vi "禹山电导率校准.vi"() -> ()   [LabVIEW 2016, in "斯坦道多参数.lvlib"]
uses:
  <vilib>/Utility/miscctls.llb/LVPointTypeDef.ctl
  <vilib>/Analysis/NI_AALBase.lvlib
  <vilib>/Analysis/NI_AALPro.lvlib
  <vilib>/Utility/config.llb/NI_LVConfig.lvlib
panel:
  out "盐度":dbl caption="盐度测量值" format="%#.2f"
  out "通讯状态":string
  out "第二点校准值":dbl
  out "第一点校准值":dbl
  out "最小值":sgl format="%.2g"
  out "最大值":sgl format="%.2g"
  in  "校准停止":bool
  in  "校准模式":u16(ring) items=["两点校准", "单点校准"]
  in  "标液2":dbl
  in  "标液1":dbl
  out "波形图表":sgl(graph) caption="历史曲线"
  out "温度测量值":dbl caption="温度" format="%#.2f"
  out "变异系数":dbl format="%.6g"
  out "standard deviation":dbl caption="标准差" format="%0.2f"
  out "mean":dbl caption="均值" format="%0.2f"
  out "提示":string
  in  "校准启动":bool
  out "测试值":dbl format="%#.2f"
  out "电极斜率":dbl format="%#.6f"
  out "电极零点":dbl format="%#.6f"
  # "电导率电极设定"
  # "℃"
  # "μS/cm"
  # "ppt"
  # "请选择校准模式:"
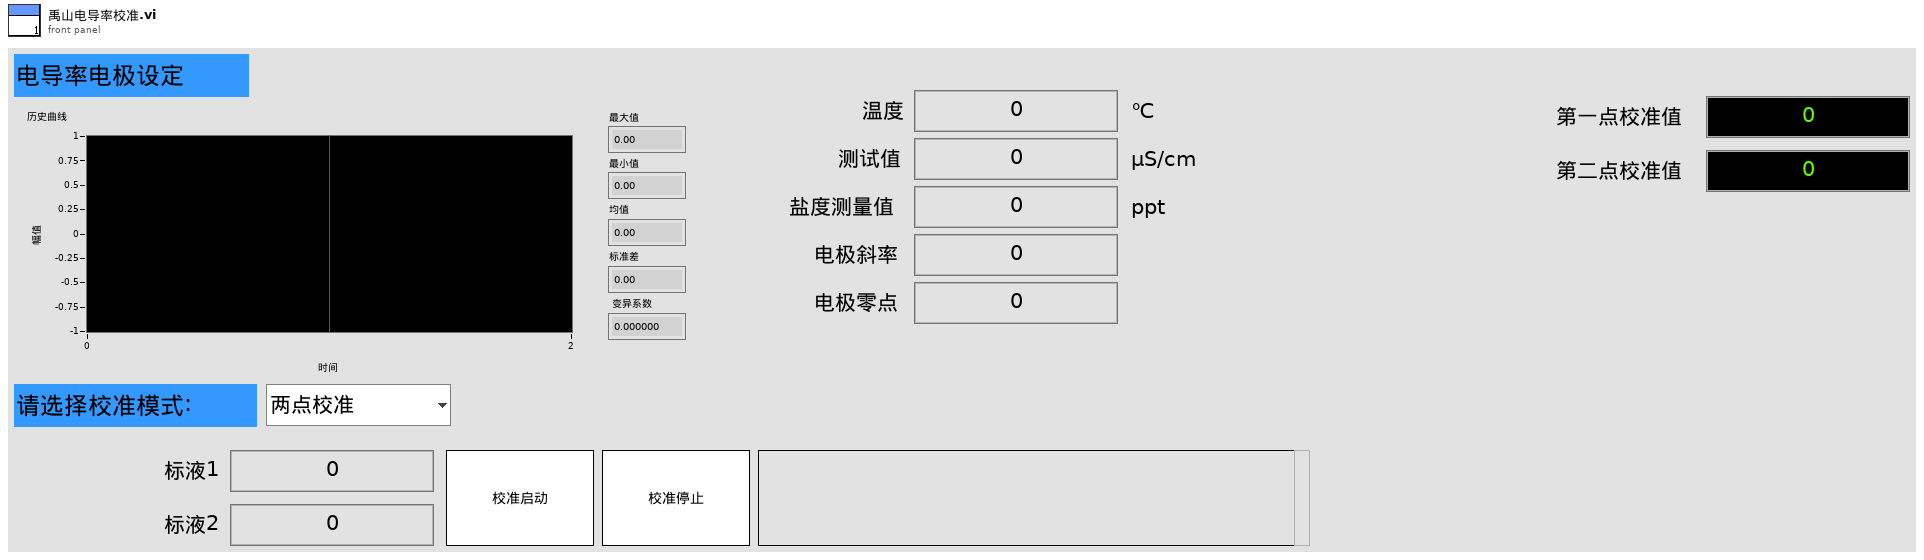
[diagram p1: front panel]
types:
  T1 = typedef "LVPointTypeDef.ctl" = cluster{"Horizontal":i16, "Vertical":i16}
  T2 = typedef "NI_LVConfig.lvlib/Config Data RefNum.ctl" = refnum<k1>
  T3 = cluster{"温度测量值":sgl, "测量值":sgl, "温度偏移修正值":sgl, "信号值":sgl}
  T4 = enum8{"Enabled", "Disabled", "Disabled and Grayed Out"}
  T5 = cluster{"ph":bool, "DO":bool, "Cond":bool, "Turb":bool, "叶绿素a":bool, "藻密度":bool, "ORP":bool}
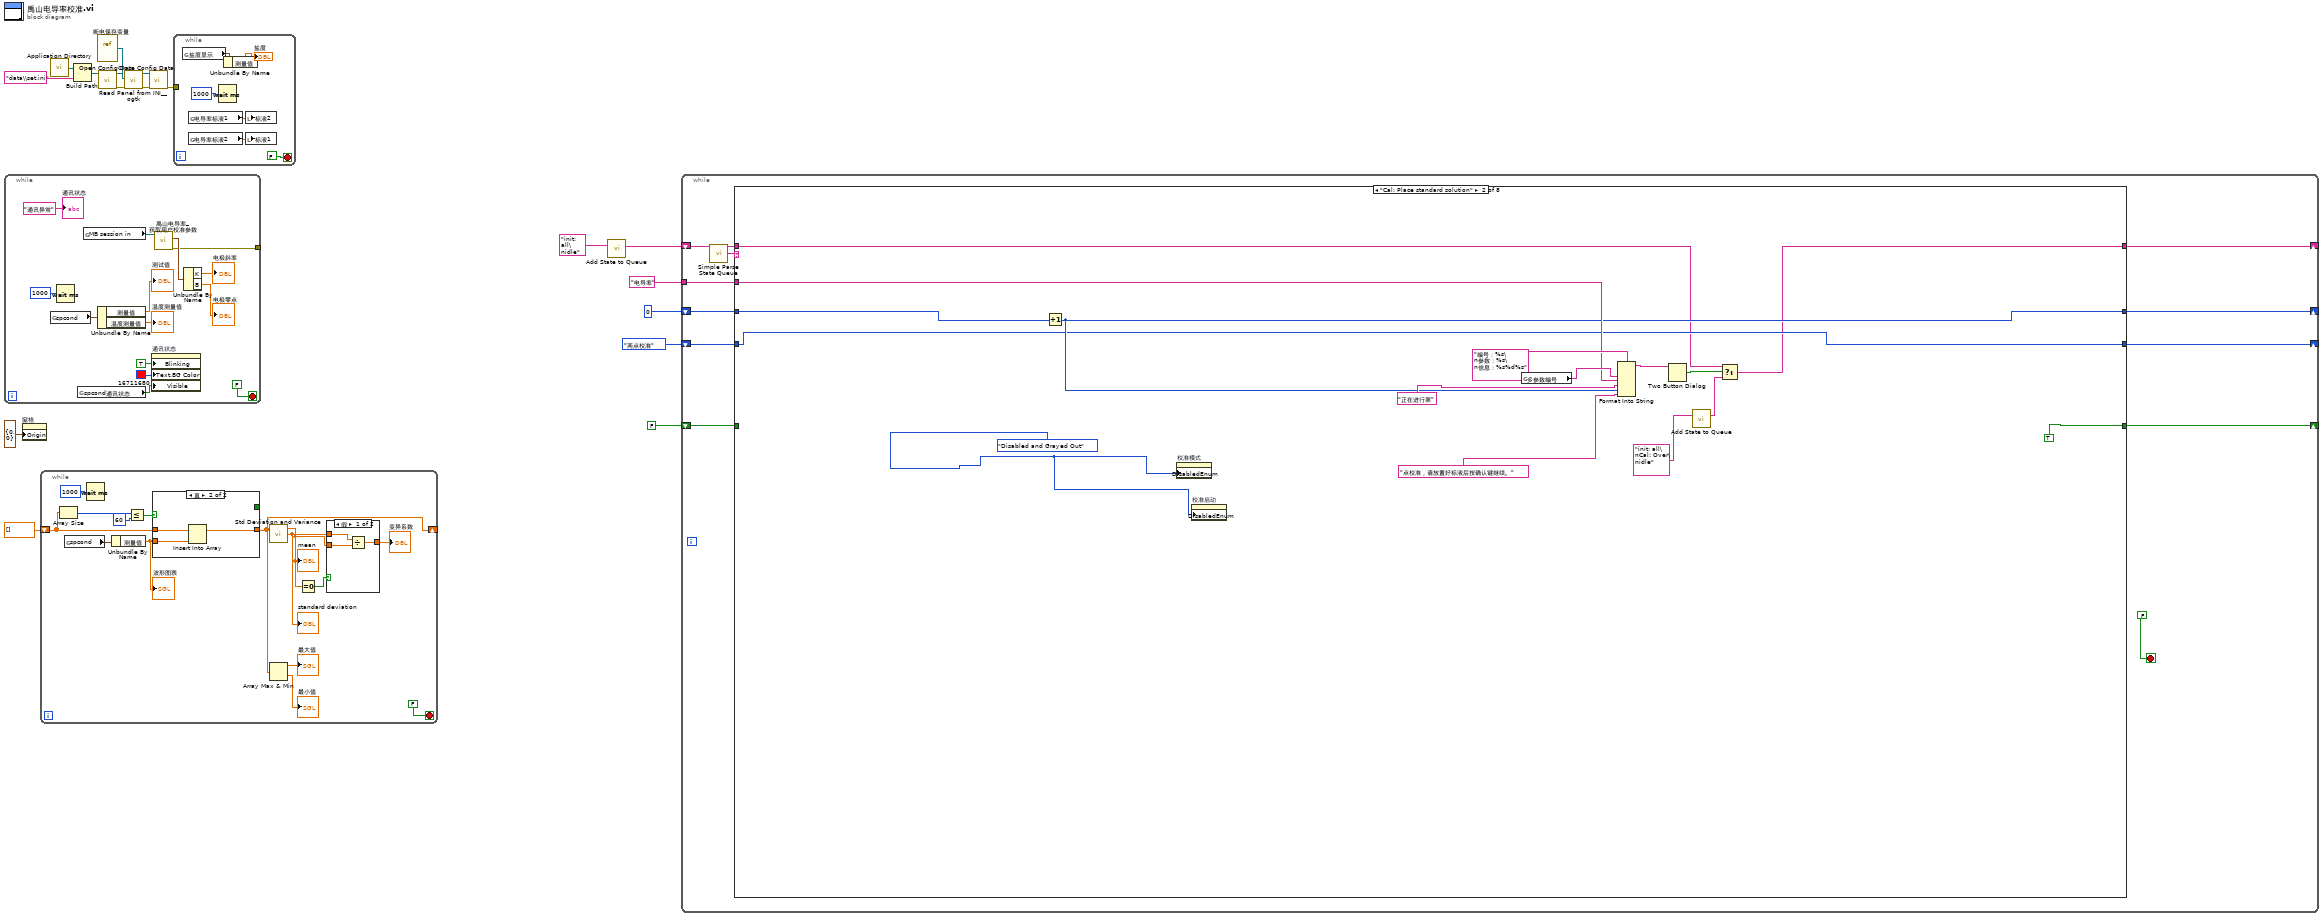
[diagram p0: block diagram]
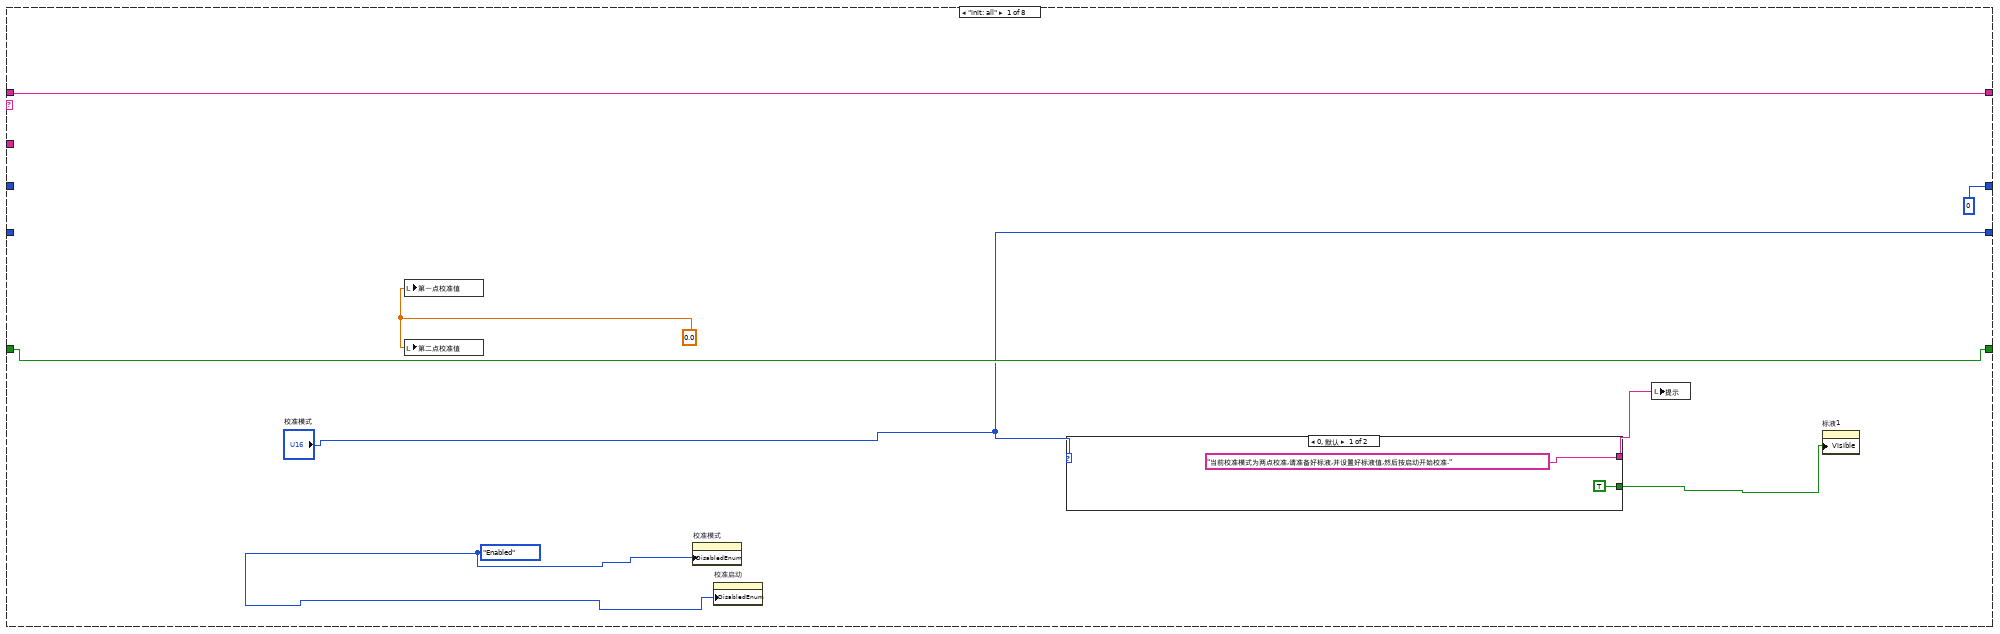
[diagram p2: hidden frame]
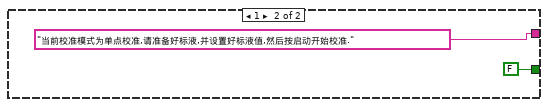
[diagram p3: hidden frame]
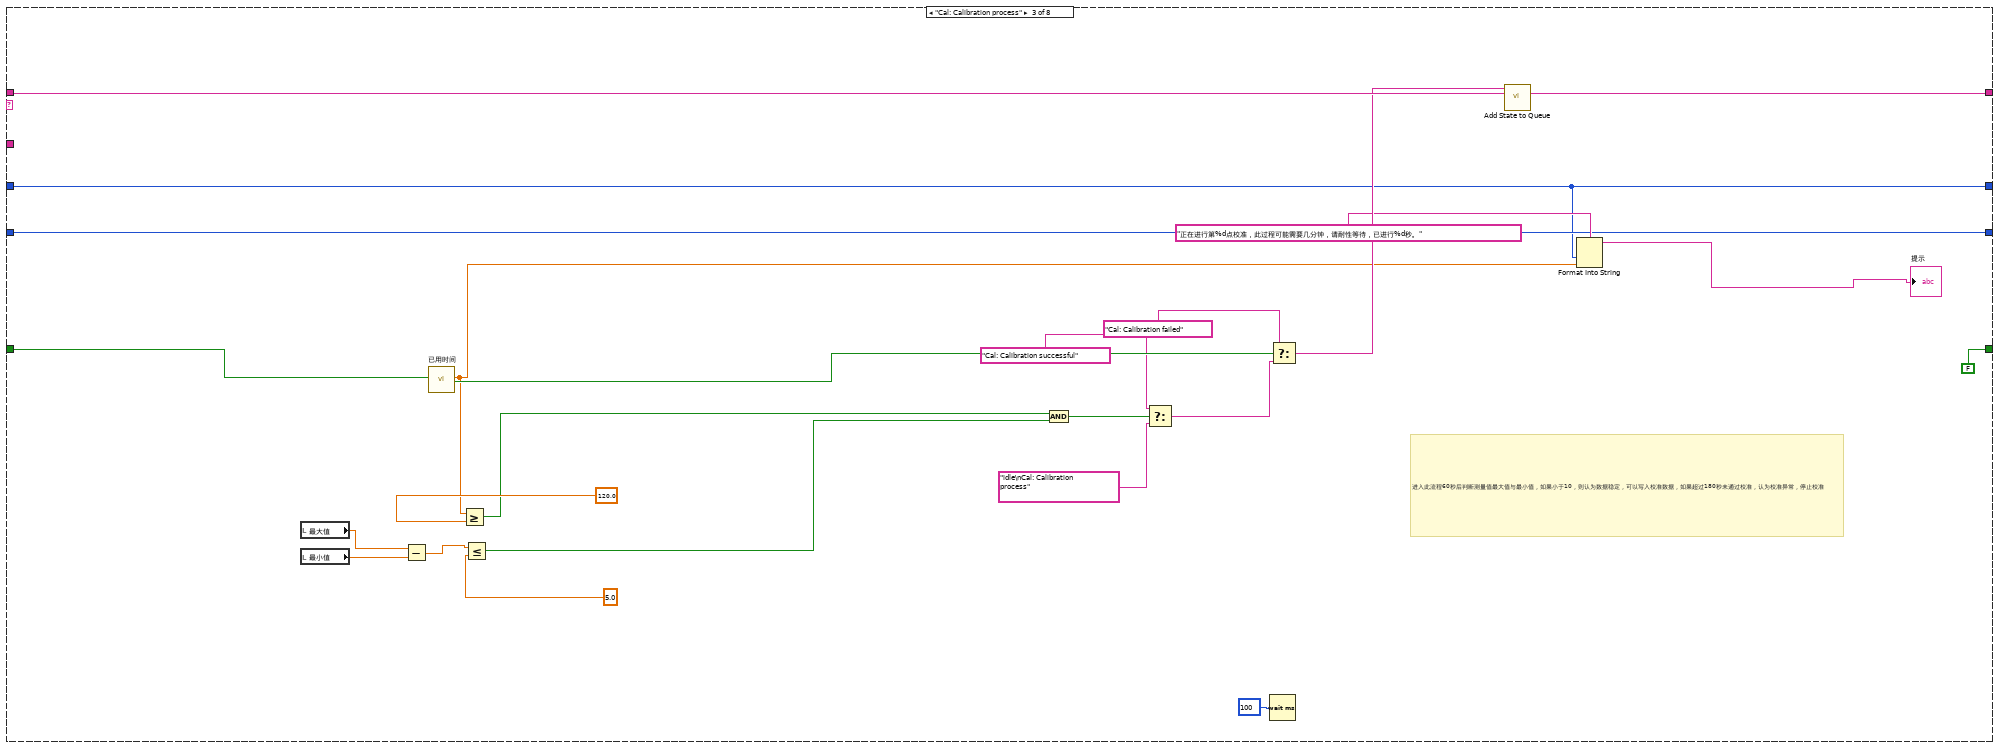
[diagram p4: hidden frame]
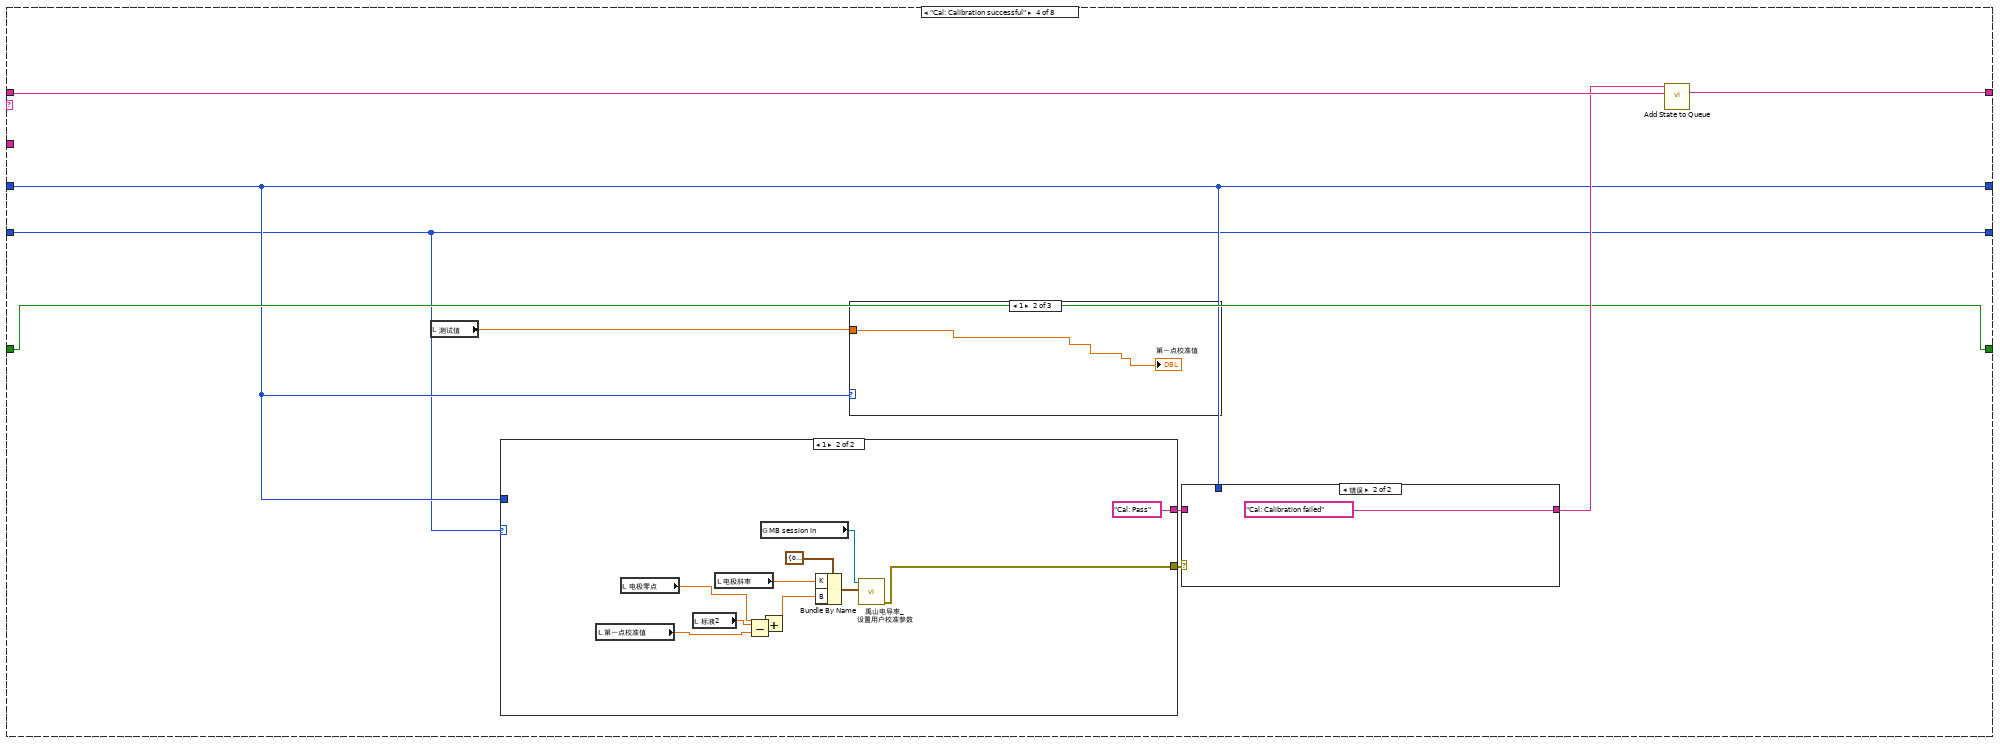
[diagram p5: hidden frame]
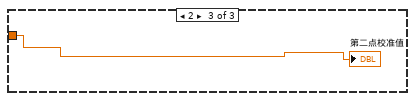
[diagram p7: hidden frame]
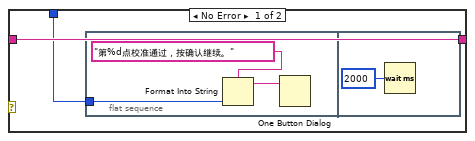
[diagram p8: hidden frame]
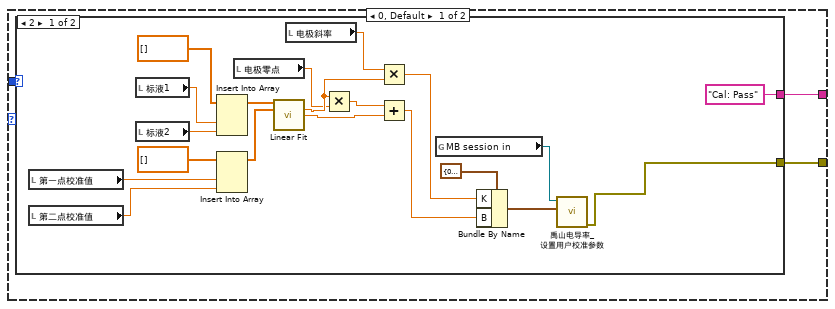
[diagram p9: hidden frame]
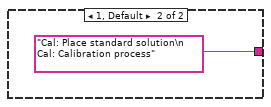
[diagram p10: hidden frame]
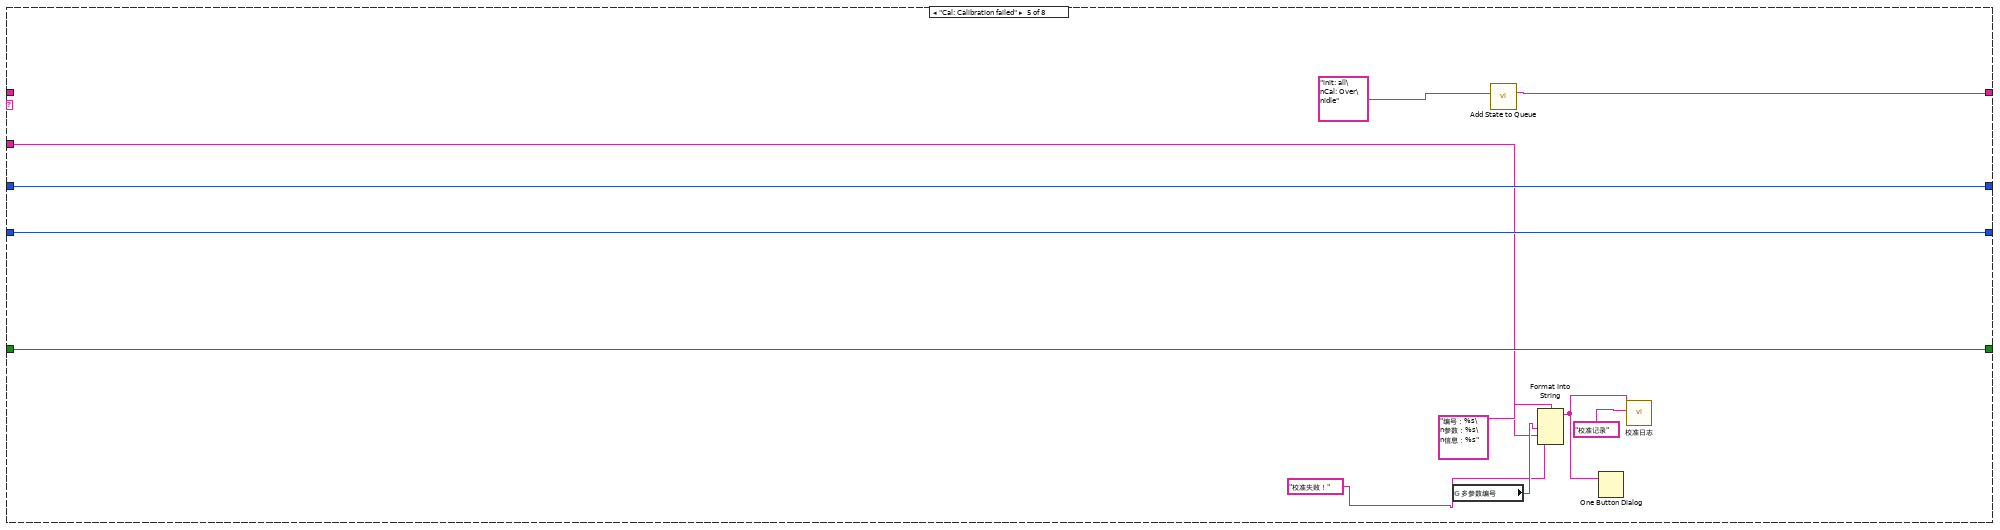
[diagram p11: hidden frame]
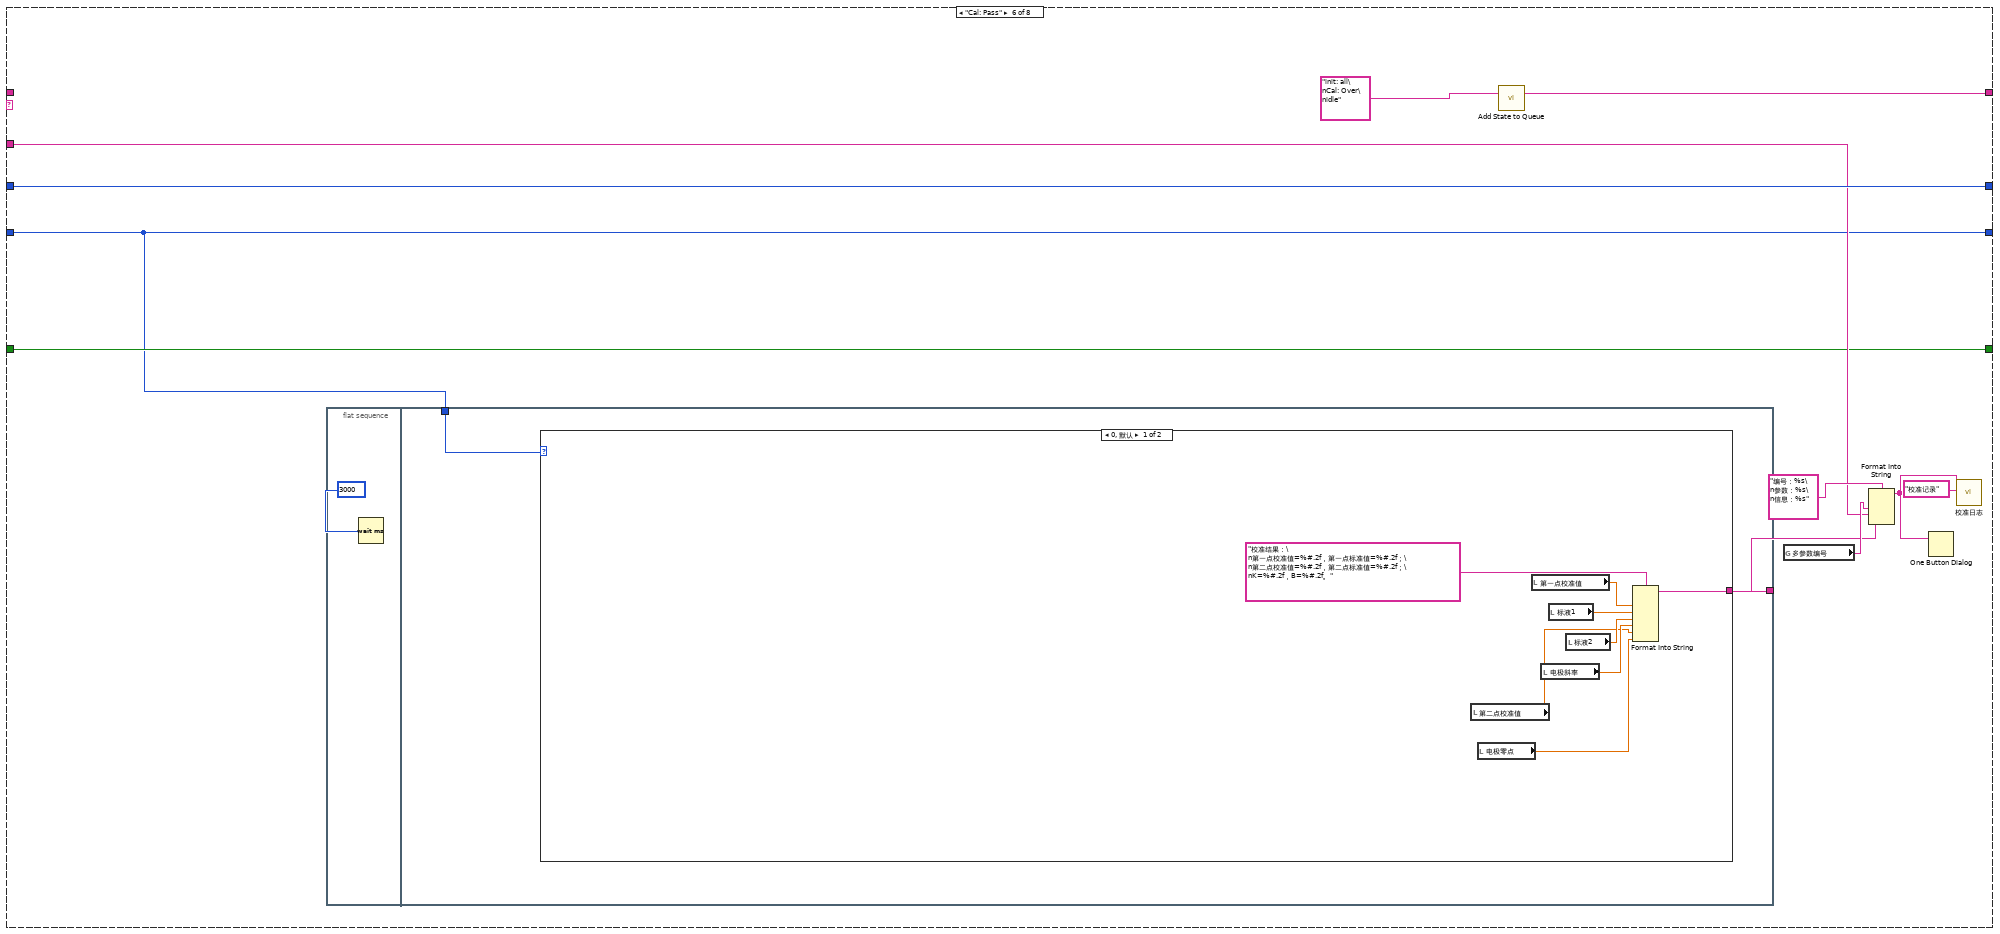
[diagram p12: hidden frame]
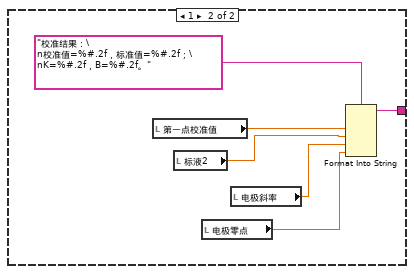
[diagram p13: hidden frame]
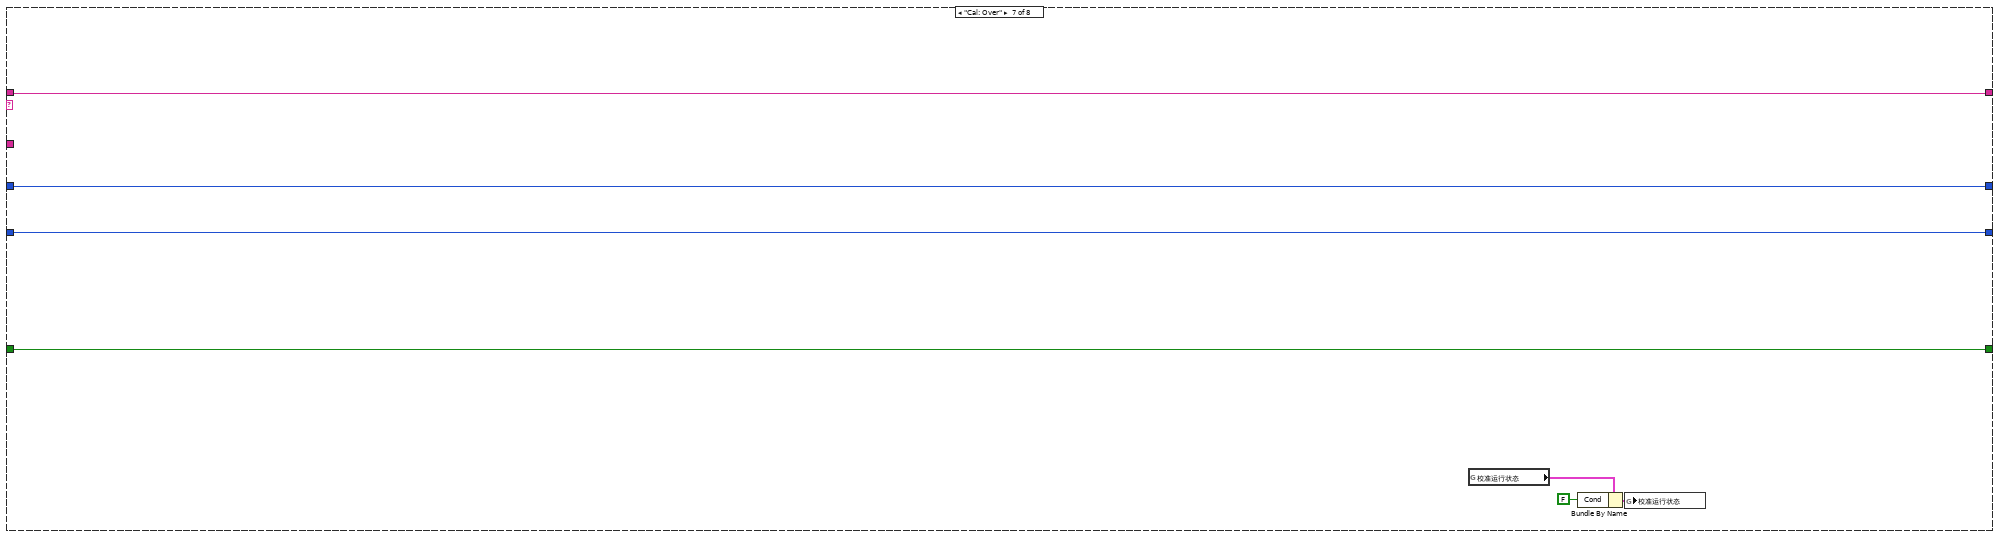
[diagram p14: hidden frame]
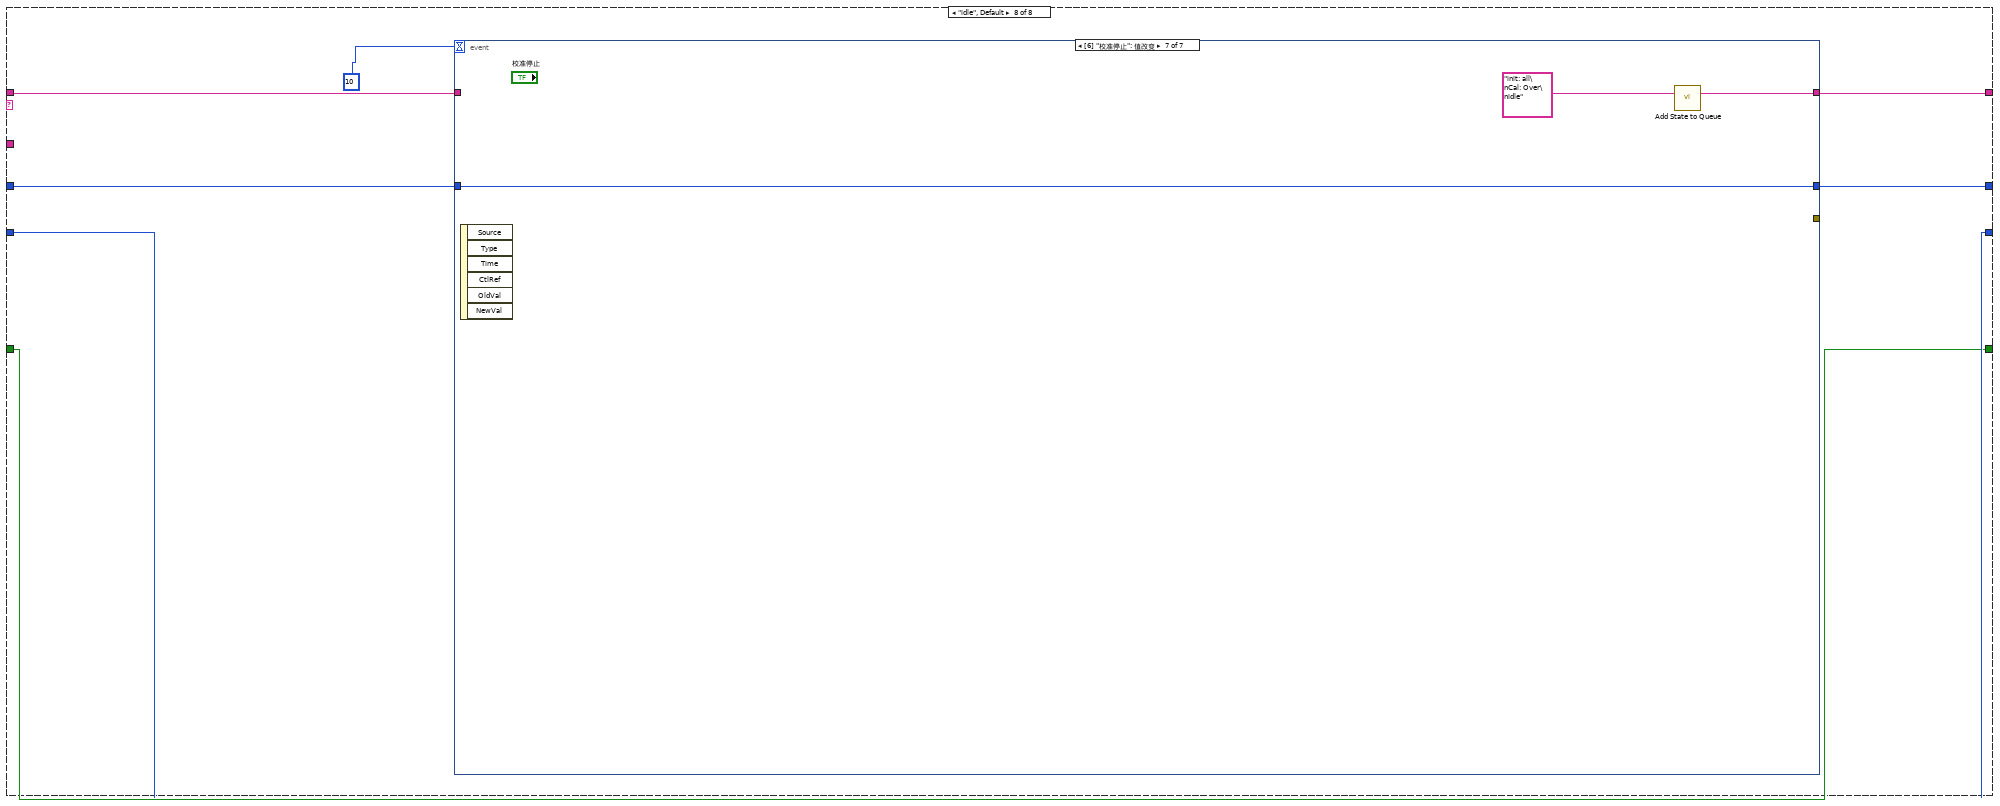
[diagram p15: hidden frame]
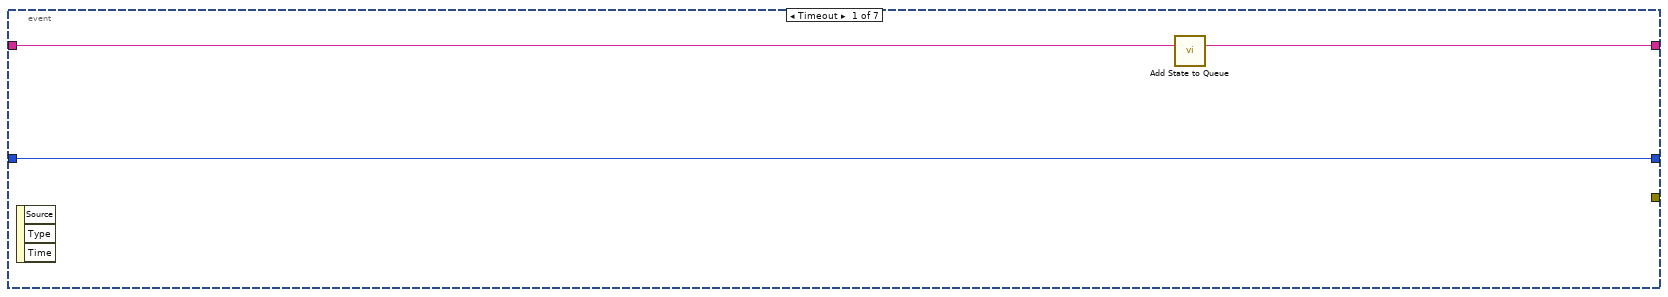
[diagram p16: hidden frame]
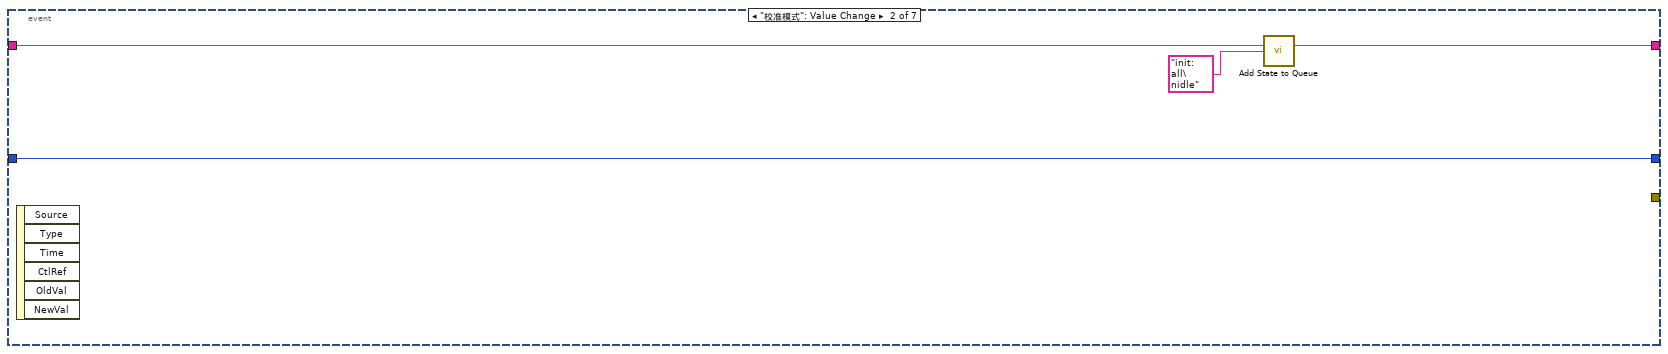
[diagram p17: hidden frame]
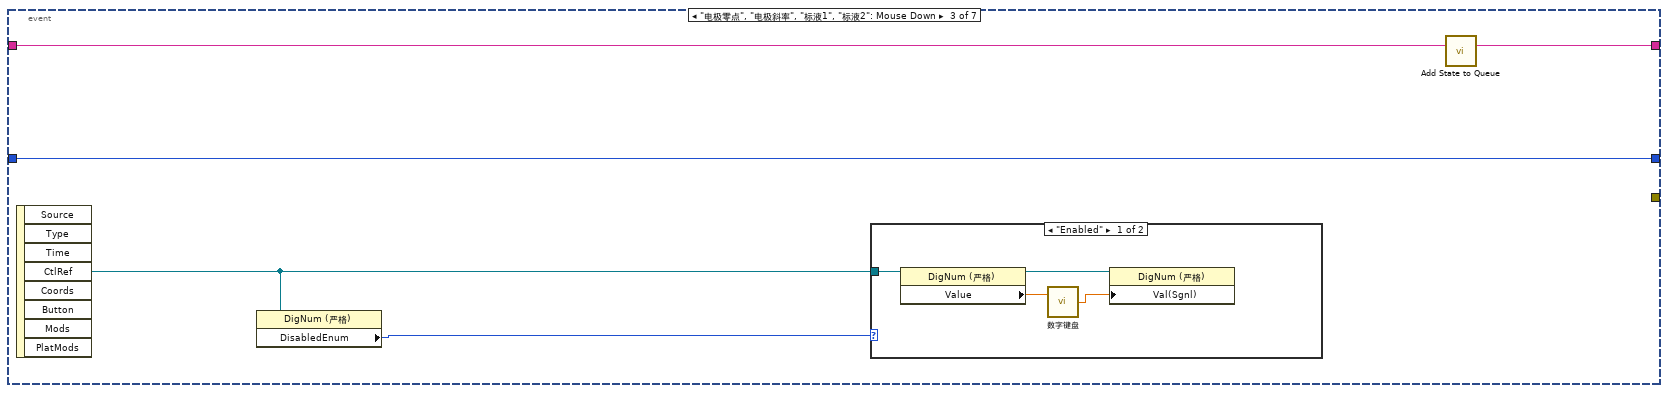
[diagram p18: hidden frame]
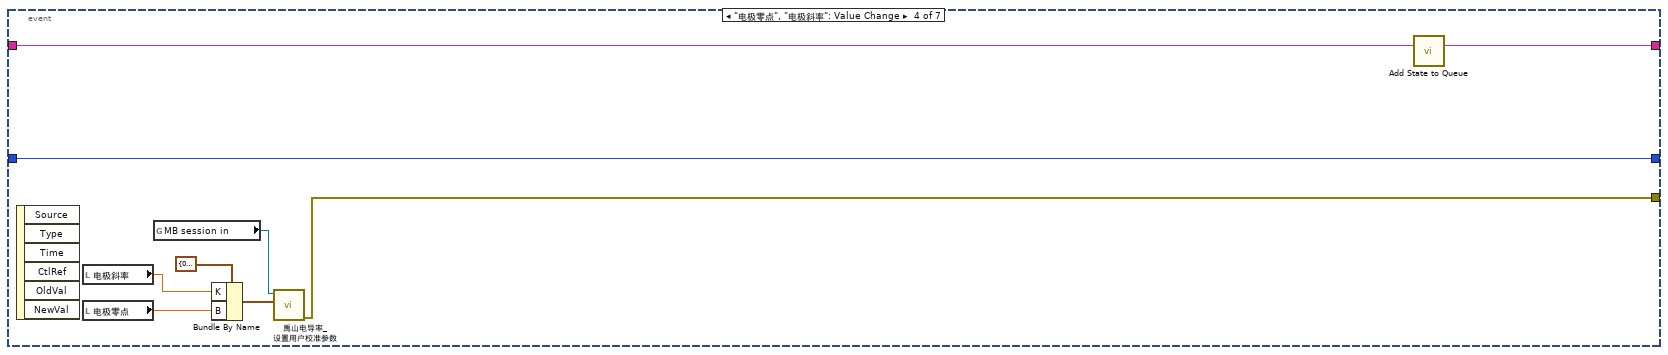
[diagram p20: hidden frame]
diagram:
  n1 = while {
    tunnel: [w26] -> _
    stop <- FALSE stop-if-true
    n2 = global read "禹山过程全局变量.vi" "spcond"() -> (w23:cluster{"温度测量值":sgl, "测量值":sgl, "错误标志":u16})
    n3 = Wait (ms)(milliseconds to wait=u32 1000 ("等待时间（毫秒）")) -> ()  [unwired: 1 out]
    n4 = global read "多参数全局变量.vi" "spcond通讯状态"() -> (w18:bool)
    n5 = global read "多参数全局变量.vi" "MB session in"() -> (w22:refnum<class "MB_Master.lvclass">)
    n6 = Unbundle By Name(w23) -> ("测量值"=→"测试值":sgl, "温度测量值"=→"温度测量值":sgl)
    n7 = property on="通讯状态" class="Str"("Blinking"=TRUE ("闪烁"), "Text.BG Color"=u32 16711680, "Visible"=w18) -> ()  [unwired: 2 in, 2 out]
    n8 = call "禹山电导率_获取用户校准参数.vi"("MB session in"=w22) -> ("error out"=w26:errorcluster, "输出值"=w29:cluster{"K":sgl, "B":sgl})  [unwired: 8 in, 1 out]
    n9 = Unbundle By Name(w29) -> ("K"=→"电极斜率":sgl, "B"=→"电极零点":sgl)
    "通讯状态" <- "通讯异常" ("当前串口")
  }
  n10 = property on="窗格" class="Pane"("Origin"=T1 {"Horizontal"=0, "Vertical"=0} ("原点")) -> ()  [unwired: 2 in, 2 out]
  n11 = while {
    shift-right: [w34] -> _
    shift-left: sgl[] [] -> [w42]
    stop <- FALSE stop-if-true
    n12 = Array Size(array=w42) -> (size(s)=w44:i32)
    n13 = global read "禹山过程全局变量.vi" "spcond"() -> (w36:cluster{"温度测量值":sgl, "测量值":sgl, "错误标志":u16})
    n14 = Wait (ms)(milliseconds to wait=u32 1000 ("等待时间（毫秒）")) -> ()  [unwired: 1 out]
    n15 = Unbundle By Name(w36) -> ("测量值"=w35:sgl)
    "波形图表" <- w35
    n16 = Less Or Equal?(x=w44, y=60) -> (x <= y?=w43:bool)
    n17 = case shown="真" w43 {
      tunnel: w42 -> [w55 w58]
      tunnel: w35 -> [w53 w57]
      tunnel: [w51 w56] -> w34
      tunnel: [TRUE _] -> _
      frame False {
        n18 = Replace Array Subset(array=w55, new element=w53) -> (w54:sgl[])  [unwired: 1 in]
        n19 = Rotate 1D Array(1:w54, 2:-1 ("n")) -> (0:w51:sgl[])
      }
      frame True {
        n20 = Insert Into Array(array=w58, new element=w57) -> (w56:sgl[])  [unwired: 1 in]
      }
    }
    n21 = call <vilib>:"Std Deviation and Variance.vi"("X"=w34) -> ("mean"=w37:dbl, "standard deviation"=w38:dbl)  [unwired: 1 in, 1 out]
    "standard deviation" <- w38
    "mean" <- w37
    n22 = Array Max & Min(array=w34) -> (max value=→"最大值":sgl, min value=→"最小值":sgl)  [unwired: 2 out]
    n23 = Equal To 0?(x=w37) -> (x = 0?=w41:bool)
    n24 = case shown="假" w41 {
      tunnel: w38 -> [w49 _]
      tunnel: [w48 _] -> w40
      tunnel: w37 -> [w47 _]
      frame False {
        n25 = Divide(x=w49, y=w47) -> (x/y=w48:dbl)
      }
      frame True {
      }
    }
    "变异系数" <- w40
  }
  n26 = call <vilib>:"Application Directory.vi"() -> ("Application Directory"=w12:path)
  n27 = Build Path(base path=w12, name or relative path="data\\set.ini" ("名称或相对路径")) -> (appended path=w13:path)
  n28 = vi-ref "断电保存变量.vi"() -> (w15:refnum<vi>)
  n29 = call <vilib>:"Open Config Data.vi"("configuration file path"=w13) -> ("error out"=w9:errorcluster, "refnum"=w8:T2)  [unwired: 8 in, 1 out]
  n30 = call <userlib>:"Read Panel from INI__ogtk.vi"("error in (no error)"=w9, "VI ref"=w15, "refnum"=w8) -> ("error out"=w11:errorcluster, "refnum out"=w10:T2)  [unwired: 7 in]
  n31 = call <vilib>:"Close Config Data.vi"("error in (no error)"=w11, "refnum"=w10) -> ("error out"=w7:errorcluster)  [unwired: 8 in, 1 out]
  n32 = while {
    tunnel: w7 -> [_]
    stop <- FALSE stop-if-true
    n33 = global read "多参数全局变量.vi" "盐度显示"() -> (w60:T3)
    n34 = global read "断电保存变量.vi" "电导率标液1"() -> (w61:dbl)
    n35 = global read "断电保存变量.vi" "电导率标液2"() -> (w62:dbl)
    n36 = Wait (ms)(milliseconds to wait=u32 1000 ("等待时间（毫秒）")) -> ()  [unwired: 1 out]
    n37 = Unbundle By Name(w60) -> ("测量值"=→"盐度":sgl)
    n38 = local write "标液2"(w61) -> ()
    n39 = local write "标液1"(w62) -> ()
  }
  n40 = call "Add State to Queue.vi"("State(s) In (\"\")"="init: all\nidle" ("State(s) In (\"\")")) -> ("States Out"=w5:string)  [unwired: 14 in]
  n41 = while {
    shift-right: [w72] -> _
    shift-left: w5 -> [w76]
    shift-right: [w69] -> _
    shift-left: 0 -> [w71]
    tunnel: "电导率" ("State(s) In (\"\")") -> [w70]
    shift-right: [w67] -> _
    shift-left: enum16{"两点校准", "单点校准"}."两点校准" ("校准模式") -> [w68]
    shift-right: [w65] -> _
    shift-left: FALSE -> [w66]
    stop <- FALSE stop-if-true
    n42 = call "Simple Parse State Queue.vi"("State Queue"=w76) -> ("Remain States"=w73:string, "Next State"=w74:string)  [unwired: 13 in]
    n43 = case shown="\"Cal: Place standard solution\"" w74 {
      tunnel: w73 -> [w84 w92 w123 w135 _ _ w224 w234]
      tunnel: [w84 w91 w122 w134 w189 w194 w224 w233] -> w72
      tunnel: w71 -> [_ w100 w107 w130 w192 w203 w223 w231]
      tunnel: w70 -> [_ w101 _ _ w183 w199 _ _]
      tunnel: [0 w98 w107 w130 w192 w203 w223 w232] -> w69
      tunnel: w68 -> [_ w97 w108 w129 w191 w195 w222 w230]
      tunnel: ["校准模式" w97 w108 w129 w191 w195 w222 w230] -> w67
      tunnel: w66 -> [w81 _ w110 w131 w190 w198 w221 w228]
      tunnel: [w81 TRUE FALSE w131 w190 w198 w221 w228] -> w65
      frame "init: all" {
        w78 = T4."Enabled" ("禁用")
        w80 = 0.0 ("第一点校准值")
        n44 = local write "第一点校准值"(w80) -> ()
        n45 = local write "第二点校准值"(w80) -> ()
        n46 = property on="校准模式" class="Ring (严格)"("DisabledEnum"=w78) -> ()  [unwired: 2 in, 2 out]
        n47 = property on="校准启动" class="Bool"("DisabledEnum"=w78) -> ()  [unwired: 2 in, 2 out]
        n48 = case shown="0, 默认" "校准模式" {
          tunnel: ["当前校准模式为两点校准,请准备好标液,并设置好标液值,然后按启动开始校准." ("提示") "当前校准模式为单点校准,请准备好标液,并设置好标液值,然后按启动开始校准." ("提示")] -> w83
          tunnel: [TRUE ("可见") FALSE ("可见")] -> w77
          frame 0, Default {
          }
          frame 1 {
          }
        }
        n49 = local write "提示"(w83) -> ()
        n50 = property on="标液1" class="DigNum (严格)"("Visible"=w77) -> ()  [unwired: 2 in, 2 out]
      }
      frame "Cal: Place standard solution" {
        w90 = T4."Disabled and Grayed Out" ("禁用")
        n51 = Increment(x=w100) -> (x+1=w98:i32)
        n52 = property on="校准模式" class="Ring (严格)"("DisabledEnum"=w90) -> ()  [unwired: 2 in, 2 out]
        n53 = property on="校准启动" class="Bool"("DisabledEnum"=w90) -> ()  [unwired: 2 in, 2 out]
        n54 = global read "多参数全局变量.vi" "多参数编号"() -> (w103:string)
        n55 = Format Into String(format string="编号：%s\n参数：%s\n信息：%s%d%s" ("格式字符串"), w103, w101, "正在进行第" ("消息"), w98, "点校准，请放置好标液后按确认键继续。" ("消息")) -> (resulting string=w95:string)  [unwired: 2 in, 1 out]
        n56 = Two Button Dialog(message=w95) -> (T button?=w94:bool)  [unwired: 2 in]
        n57 = call "Add State to Queue.vi"("State(s) In (\"\")"="init: all\nCal: Over\nidle" ("State(s) In (\"\")")) -> ("States Out"=w93:string)  [unwired: 14 in]
        n58 = Select(t=w92, s=w94, f=w93) -> (s? t:f=w91:string)
      }
      frame "Cal: Calibration process" {
        # "进入此流程60秒后判断测量值最大值与最小值，如果小于10，则认为数据稳定，可以写入校准数据，如果超过180秒未通过校准，认为校准异常，停止校准"
        n59 = local read "最大值"() -> (w127:sgl)
        n60 = local read "最小值"() -> (w126:sgl)
        n61 = Subtract(x=w127, y=w126) -> (x-y=w128:sgl)
        n62 = call "已用时间"("Reset"=w110) -> ("Elapsed Time (s)"=w106:dbl, "Time has Elapsed"=w124:bool)  [unwired: 11 in, 6 out]
        n63 = Greater Or Equal?(x=w106, y=120.0) -> (x >= y?=w119:bool)
        n64 = Less Or Equal?(x=w128, y=5.0) -> (x <= y?=w115:bool)
        n65 = And(x=w119, y=w115) -> (x .and. y?=w116:bool)
        n66 = Select(t="Cal: Calibration successful" ("State(s) In (\"\")"), s=w116, f="idle\nCal: Calibration process" ("State(s) In (\"\")")) -> (s? t:f=w114:string)
        n67 = Wait (ms)(milliseconds to wait=u32 100 ("等待时间（毫秒）")) -> ()  [unwired: 1 out]
        n68 = Select(t="Cal: Calibration failed" ("State(s) In (\"\")"), s=w124, f=w114) -> (s? t:f=w113:string)
        n69 = call "Add State to Queue.vi"("State(s) In Front (\"\")"=w113, "State(s) In (\"\")"=w123) -> ("States Out"=w122:string)  [unwired: 13 in]
        n70 = Format Into String(format string="正在进行第%d点校准，此过程可能需要几分钟，请耐性等待，已进行%d秒。" ("格式字符串"), w107, w106) -> (resulting string=→"提示":string)  [unwired: 2 in, 1 out]
      }
      frame "Cal: Calibration successful" {
        n71 = local read "测试值"() -> (w132:dbl)
        n72 = case shown="1" w129 {
          tunnel: [w149 w171] -> w137
          tunnel: [w148 "Cal: Pass" ("State(s) In (\"\")")] -> w136
          tunnel: w130 -> [w147 _]
          frame 0, Default {
            n73 = case shown="2" w147 {
              tunnel: [w150 _] -> w149
              tunnel: ["Cal: Pass" ("State(s) In (\"\")") "Cal: Place standard solution\n Cal: Calibration process" ("State(s) In (\"\")")] -> w148
              frame 2 {
                n74 = local read "第一点校准值"() -> (w167:dbl)
                n75 = local read "第二点校准值"() -> (w166:dbl)
                n76 = local read "标液1"() -> (w164:dbl)
                n77 = local read "标液2"() -> (w163:dbl)
                n78 = Insert Into Array(array=dbl[] [] ("Weight"), new element #1=w164, new element #2=w163) -> (w162:dbl[])  [unwired: 1 in]
                n79 = Insert Into Array(array=dbl[] [] ("Weight"), new element #1=w167, new element #2=w166) -> (w161:dbl[])  [unwired: 1 in]
                n80 = local read "电极零点"() -> (w154:dbl)
                n81 = call <vilib>:"Linear Fit.vi"("Y"=w162, "X"=w161) -> ("slope"=w155:dbl, "intercept"=w152:dbl)  [unwired: 9 in, 3 out]
                n82 = local read "电极斜率"() -> (w157:dbl)
                n83 = Multiply(x=w155, y=w154) -> (x*y=w153:dbl)
                n84 = Multiply(x=w157, y=w155) -> (x*y=w156:dbl)
                n85 = Add(x=w153, y=w152) -> (x+y=w151:dbl)
                n86 = global read "多参数全局变量.vi" "MB session in"() -> (w160:refnum<class "MB_Master.lvclass">)
                n87 = Bundle By Name(cluster=cluster{"K":sgl, "B":sgl} {"K"=0.0, "B"=0.0} ("用户校准参数"), "K"=w156, "B"=w151) -> (w159:cluster{"K":sgl, "B":sgl})
                n88 = call "禹山电导率_设置用户校准参数.vi"("用户校准参数"=w159, "MB session in"=w160) -> ("error out"=w150:errorcluster)  [unwired: 8 in, 1 out]
              }
              frame 1, Default {
              }
            }
          }
          frame 1 {
            n89 = local read "第一点校准值"() -> (w176:dbl)
            n90 = local read "电极零点"() -> (w172:dbl)
            n91 = local read "标液2"() -> (w175:dbl)
            n92 = local read "电极斜率"() -> (w177:dbl)
            n93 = Subtract(x=w175, y=w176) -> (x-y=w174:dbl)
            n94 = global read "多参数全局变量.vi" "MB session in"() -> (w180:refnum<class "MB_Master.lvclass">)
            n95 = Add(x=w172, y=w174) -> (x+y=w173:dbl)
            n96 = Bundle By Name(cluster=cluster{"K":sgl, "B":sgl} {"K"=0.0, "B"=0.0} ("用户校准参数"), "K"=w177, "B"=w173) -> (w179:cluster{"K":sgl, "B":sgl})
            n97 = call "禹山电导率_设置用户校准参数.vi"("用户校准参数"=w179, "MB session in"=w180) -> ("error out"=w171:errorcluster)  [unwired: 8 in, 1 out]
          }
        }
        n98 = case shown="1" w130 {
          tunnel: w132 -> [_ w138 w139]
          frame 0, Default {
          }
          frame 1 {
            "第一点校准值" <- w138
          }
          frame 2 {
            "第二点校准值" <- w139
          }
        }
        n99 = case shown="错误" w137 {
          tunnel: w136 -> [w141 _]
          tunnel: [w141 "Cal: Calibration failed" ("State(s) In (\"\")")] -> w133
          tunnel: w130 -> [w140 _]
          frame No Error {
            n100 = flat-sequence {
              tunnel: w140 -> [w142]
              frame #0 {
                n101 = Format Into String(format string="第%d点校准通过，按确认继续。" ("格式字符串"), w142) -> (resulting string=w144:string)  [unwired: 2 in, 1 out]
                n102 = One Button Dialog(message=w144) -> ()  [unwired: 1 in, 1 out]
              }
              frame #1 {
                n103 = Wait (ms)(milliseconds to wait=u32 2000 ("等待时间（毫秒）")) -> ()  [unwired: 1 out]
              }
            }
          }
          frame Error {
          }
        }
        n104 = call "Add State to Queue.vi"("State(s) In Front (\"\")"=w133, "State(s) In (\"\")"=w135) -> ("States Out"=w134:string)  [unwired: 13 in]
      }
      frame "Cal: Calibration failed" {
        n105 = global read "多参数全局变量.vi" "多参数编号"() -> (w186:string)
        n106 = call "Add State to Queue.vi"("State(s) In (\"\")"="init: all\nCal: Over\nidle" ("State(s) In (\"\")")) -> ("States Out"=w189:string)  [unwired: 14 in]
        n107 = Format Into String(format string="编号：%s\n参数：%s\n信息：%s" ("格式字符串"), w186, w183, "校准失败！" ("消息")) -> (resulting string=w185:string)  [unwired: 2 in, 1 out]
        n108 = One Button Dialog(message=w185) -> ()  [unwired: 1 in, 1 out]
        n109 = call "校准日志.vi"("table"="校准记录", "日志信息"=w185) -> ()  [unwired: 9 in, 1 out]
      }
      frame "Cal: Pass" {
        n110 = flat-sequence {
          tunnel: [w206] -> w196
          tunnel: w195 -> [w205]
          frame #0 {
            n111 = Wait (ms)(milliseconds to wait=u32 3000 ("等待时间（毫秒）")) -> ()  [unwired: 1 out]
          }
          frame #1 {
            n112 = case shown="0, 默认" w205 {
              tunnel: [w214 w220] -> w206
              frame 0, Default {
                n113 = local read "第二点校准值"() -> (w208:dbl)
                n114 = local read "电极零点"() -> (w207:dbl)
                n115 = local read "第一点校准值"() -> (w212:dbl)
                n116 = local read "电极斜率"() -> (w209:dbl)
                n117 = local read "标液1"() -> (w213:dbl)
                n118 = local read "标液2"() -> (w210:dbl)
                n119 = Format Into String(format string="校准结果：\n第一点校准值=%#.2f，第一点标准值=%#.2f；\n第二点校准值=%#.2f，第二点标准值=%#.2f；\nK=%#.2f，B=%#.2f。" ("提示"), w212, w213, w210, w209, w208, w207) -> (resulting string=w214:string)  [unwired: 2 in, 1 out]
              }
              frame 1 {
                n120 = local read "第一点校准值"() -> (w219:dbl)
                n121 = local read "标液2"() -> (w217:dbl)
                n122 = local read "电极零点"() -> (w215:dbl)
                n123 = local read "电极斜率"() -> (w216:dbl)
                n124 = Format Into String(format string="校准结果：\n校准值=%#.2f，标准值=%#.2f；\nK=%#.2f，B=%#.2f。" ("提示"), w219, w217, w216, w215) -> (resulting string=w220:string)  [unwired: 2 in, 1 out]
              }
            }
          }
        }
        n125 = call "Add State to Queue.vi"("State(s) In (\"\")"="init: all\nCal: Over\nidle" ("State(s) In (\"\")")) -> ("States Out"=w194:string)  [unwired: 14 in]
        n126 = global read "多参数全局变量.vi" "多参数编号"() -> (w200:string)
        n127 = Format Into String(format string="编号：%s\n参数：%s\n信息：%s" ("格式字符串"), w200, w199, w196) -> (resulting string=w197:string)  [unwired: 2 in, 1 out]
        n128 = One Button Dialog(message=w197) -> ()  [unwired: 1 in, 1 out]
        n129 = call "校准日志.vi"("table"="校准记录", "日志信息"=w197) -> ()  [unwired: 9 in, 1 out]
      }
      frame "Cal: Over" {
        n130 = global read "多参数全局变量.vi" "校准运行状态"() -> (w226:T5)
        n131 = Bundle By Name(cluster=w226, "Cond"=FALSE) -> (w227:T5)
        n132 = global write "多参数全局变量.vi" "校准运行状态"(w227) -> ()
      }
      frame "idle", Default {
        n133 = event shown="[6] \"校准停止\": 值改变" {
          selector: _ -> [_ _ _ _ _ _ _]
          dyn-events: _ -> [_ _ _ _ _ _ _]
          timeout: 10 -> [_ _ _ _ _ _ _]
          tunnel: [_ _ _ w252 _ _ _] -> _
          tunnel: w234 -> [w237 w241 w244 w251 w260 w285 _]
          tunnel: [w236 w240 w245 w258 w261 w284 w287] -> w233
          tunnel: [w235 w238 w246 w259 w262 w282 w288] -> w232
          tunnel: w231 -> [w235 w238 w246 w259 w262 w282 w288]
          event Timeout {
            n134 = event-data() -> ()  [unwired: 1 in, 3 out]
            n135 = call "Add State to Queue.vi"("State(s) In (\"\")"=w237) -> ("States Out"=w236:string)  [unwired: 14 in]
          }
          event "校准模式": Value Change {
            n136 = event-data() -> ()  [unwired: 1 in, 6 out]
            n137 = call "Add State to Queue.vi"("State(s) In (\"\")"=w241, "State(s) At Back (\"\")"="init: all\nidle" ("State(s) In (\"\")")) -> ("States Out"=w240:string)  [unwired: 13 in]
          }
          event "电极零点", "电极斜率", "标液1", "标液2": Mouse Down {
            n138 = event-data() -> ("CtlRef"=w243:refnum<vi>)  [unwired: 1 in, 7 out]
            n139 = property class="DigNum (严格)"(reference=w243) -> ("DisabledEnum"=w242:T4)  [unwired: 1 in, 2 out]
            n140 = case shown="\"Enabled\"" w242 {
              tunnel: w243 -> [w250 _]
              frame "Enabled" {
                n141 = property class="DigNum (严格)"(reference=w250) -> (reference out=w247:refnum<vi>, "Value"=w248:dbl)  [unwired: 1 in, 1 out]
                n142 = call "数字键盘.vi"("OldNumber"=w248) -> ("NewNumber"=w249:dbl)  [unwired: 1 in]
                n143 = property class="DigNum (严格)"(reference=w247, "Val(Sgnl)"=w249) -> ()  [unwired: 1 in, 2 out]
              }
              frame "Disabled", Default {
              }
            }
            n144 = call "Add State to Queue.vi"("State(s) In (\"\")"=w244) -> ("States Out"=w245:string)  [unwired: 14 in]
          }
          event "电极零点", "电极斜率": Value Change {
            n145 = event-data() -> ()  [unwired: 1 in, 6 out]
            n146 = local read "电极斜率"() -> (w255:dbl)
            n147 = local read "电极零点"() -> (w254:dbl)
            n148 = global read "多参数全局变量.vi" "MB session in"() -> (w253:refnum<class "MB_Master.lvclass">)
            n149 = Bundle By Name(cluster=cluster{"K":sgl, "B":sgl} {"K"=0.0, "B"=0.0} ("用户校准参数"), "K"=w255, "B"=w254) -> (w256:cluster{"K":sgl, "B":sgl})
            n150 = call "禹山电导率_设置用户校准参数.vi"("用户校准参数"=w256, "MB session in"=w253) -> ("error out"=w252:errorcluster)  [unwired: 8 in, 1 out]
            n151 = call "Add State to Queue.vi"("State(s) In (\"\")"=w251) -> ("States Out"=w258:string)  [unwired: 14 in]
          }
          event "标液1", "标液2": Value Change {
            n152 = event-data() -> ()  [unwired: 1 in, 6 out]
            n153 = flat-sequence {
              frame #0 {
                n154 = global write "断电保存变量.vi" "电导率标液1"("标液2") -> ()
                n155 = global write "断电保存变量.vi" "电导率标液2"("标液1") -> ()
              }
              frame #1 {
                n156 = call <vilib>:"Application Directory.vi"() -> ("Application Directory"=w274:path)
                n157 = Build Path(base path=w274, name or relative path="data\\set.ini" ("名称或相对路径")) -> (appended path=w273:path)
                n158 = call <vilib>:"Open Config Data.vi"("configuration file path"=w273) -> ("error out"=w277:errorcluster, "refnum"=w278:T2)  [unwired: 8 in, 1 out]
                n159 = vi-ref "断电保存变量.vi"() -> (w271:refnum<vi>)
                n160 = call <userlib>:"Write Panel to INI__ogtk.vi"("error in (no error)"=w277, "VI ref"=w271, "refnum"=w278) -> ("error out"=w275:errorcluster, "refnum out"=w276:T2)  [unwired: 7 in]
                n161 = call <vilib>:"Close Config Data.vi"("error in (no error)"=w275, "refnum"=w276) -> ("error out"=w267:errorcluster, "file path"=w268:path)  [unwired: 8 in]
                n162 = Open/Create/Replace File(file path (use dialog)=w268, error in=w267) -> (refnum out=w269:refnum<file>, error out=w270:errorcluster)  [unwired: 4 in, 1 out]
                n163 = Flush File(refnum=w269, error in=w270) -> (refnum out=w265:refnum<file>, error out=w266:errorcluster)
                n164 = Close File(refnum=w265, error in=w266) -> ()  [unwired: 2 out]
              }
            }
            n165 = call "Add State to Queue.vi"("State(s) In (\"\")"=w260) -> ("States Out"=w261:string)  [unwired: 14 in]
          }
          event "校准启动": Value Change {
            n166 = event-data() -> ()  [unwired: 1 in, 6 out]
            n167 = global read "多参数全局变量.vi" "校准运行状态"() -> (w280:T5)
            n168 = Bundle By Name(cluster=w280, "Cond"=TRUE) -> (w281:T5)
            n169 = call "Add State to Queue.vi"("State(s) In (\"\")"=w285, "State(s) At Back (\"\")"="init: all\nCal: Place standard solution\n Cal: Calibration process\nidle" ("State(s) In (\"\")")) -> ("States Out"=w284:string)  [unwired: 13 in]
            n170 = global write "多参数全局变量.vi" "校准运行状态"(w281) -> ()
          }
          event "校准停止": Value Change {
            n171 = event-data() -> ()  [unwired: 1 in, 6 out]
            n172 = call "Add State to Queue.vi"("State(s) In (\"\")"="init: all\nCal: Over\nidle" ("State(s) In (\"\")")) -> ("States Out"=w287:string)  [unwired: 14 in]
          }
        }
      }
    }
  }
